vi "Labview_USB_I2C_AT24C02_SCTL.vi"() -> ()   [LabVIEW 2010]
uses:
  Labview_USB_I2C_AM2321B/lib/labview_32bit/ControlI2C/Ginkgo_Driver.dll
panel:
  out "Flag(T:read;F:write)":bool=TRUE
  in  "Constant":T1={"DevType"=1, "DevIndex"=0, "I2CIndex"=0, "Addr"=0, "SubAddr"=0}
  in  "pInitConfig":T2={"MasterMode"=1, "ControlMode"=1, "AddrType"=7, "SubAddrWidth"=0, "Addr"=0, "@dummy control@"=0, "@dummy control@"=0, "ClockSpeed"=0}
  in  "pTimeConfig":T3
  out "error out":errorcluster
  in  "Read":bool
  in  "Write":bool
  in  "Sub Addr(Hex)":u8 format="%x"
  in  "Slave Addr(Hex)":u8 format="%x"
  out "Read Data(Hex)":string
  in  "Channel Index":u16(ring) items=["0", "1"]
  in  "Speed":u32(ring)=800000 items=["800Kbps"=800000, "400Kbps"=400000, "200Kbps"=200000, "100Kbps"=100000, "50Kbps"=50000]
  in  "Write Data(Hex)":string
  in  "Device Index":u16(ring) items=["0", "1", "2", "3", "4", "5", "6", "7", "8", "9"]
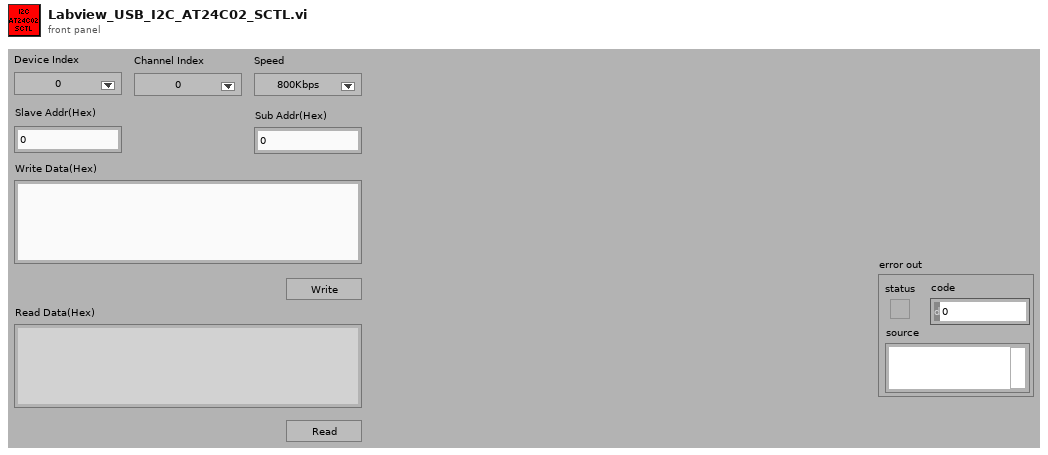
[diagram p1: front panel]
types:
  T1 = cluster{"DevType":i32, "DevIndex":i32, "I2CIndex":i32, "Addr":u16, "SubAddr":u32}
  T2 = cluster{"MasterMode":u8, "ControlMode":u8, "AddrType":u8, "SubAddrWidth":u8, "Addr":u16, "@dummy control@":i8, "@dummy control@":i8, "ClockSpeed":u32}
  T3 = cluster{"tHD_STA":u16, "tSU_STA":u16, "tLOW":u16, "tHIGH":u16, "tSU_DAT":u16, "tSU_STO":u16, "tDH":u16, "tDH_DAT":u16, "tAA":u16, "tR":u16, "tF":u16, "tBuf":u16, "tACK[0]":u8, "tACK[1]":u8, "tACK[2]":u8, "tACK[3]":u8, "tStart":u16, "tStop":u16}
  T4 = enum16{"Init", "Write", "Read", "Idel", "Close", "Error"}
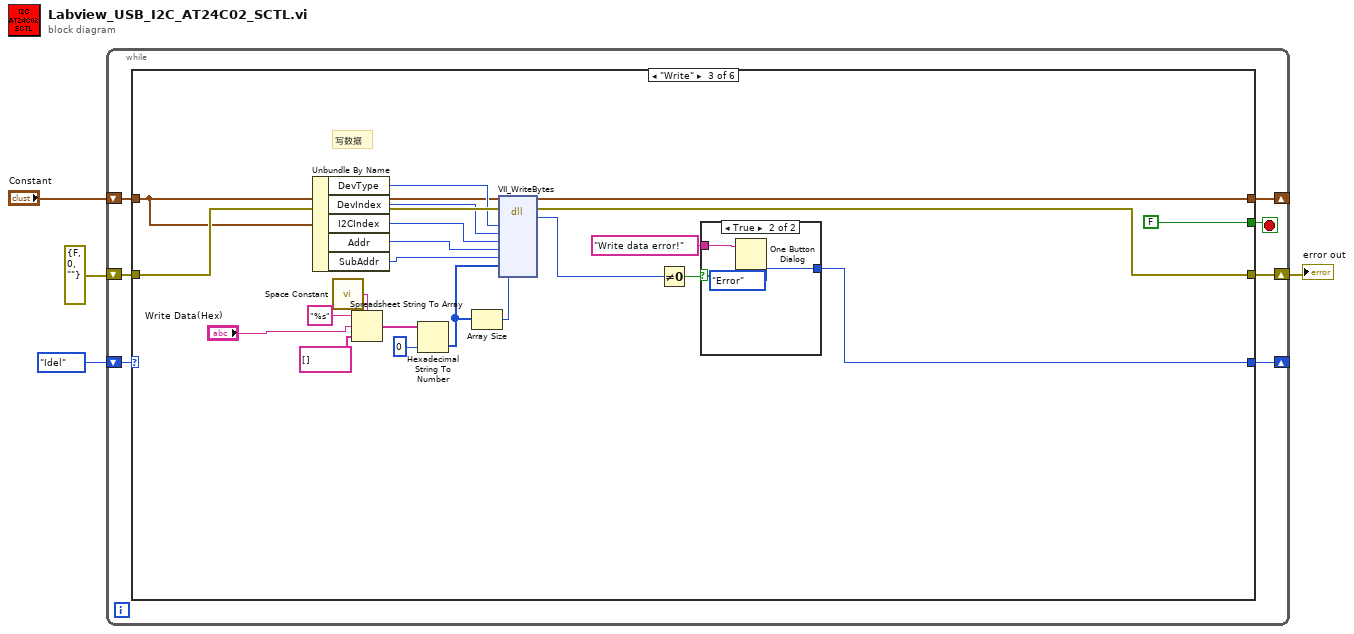
[diagram p0: block diagram]
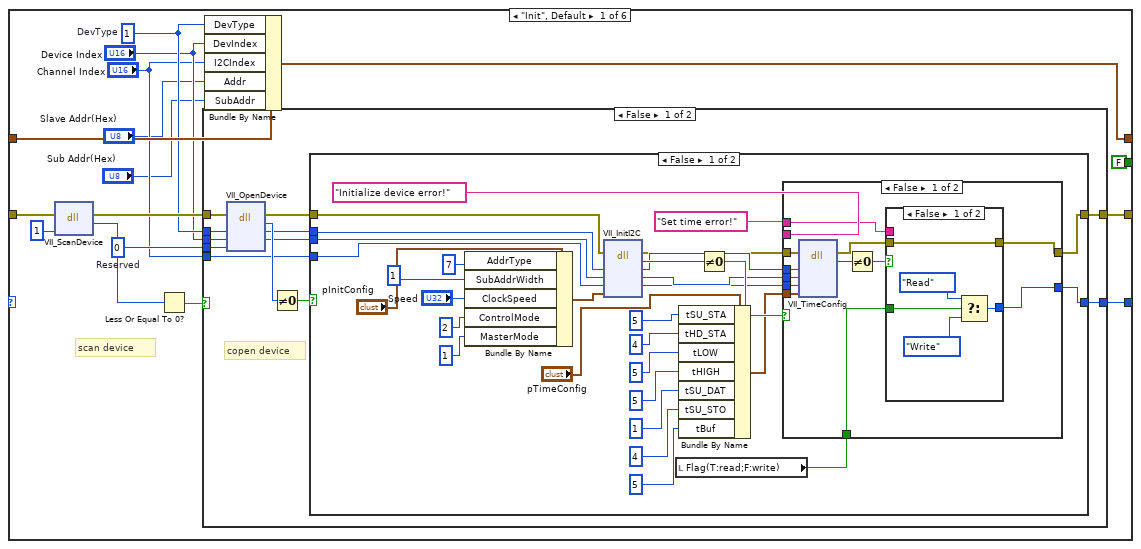
[diagram p2: hidden frame]
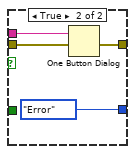
[diagram p3: hidden frame]
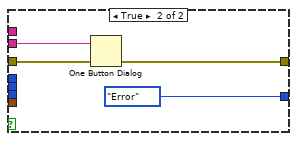
[diagram p4: hidden frame]
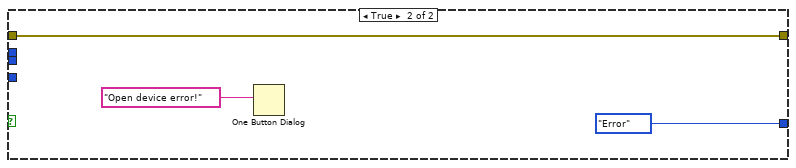
[diagram p5: hidden frame]
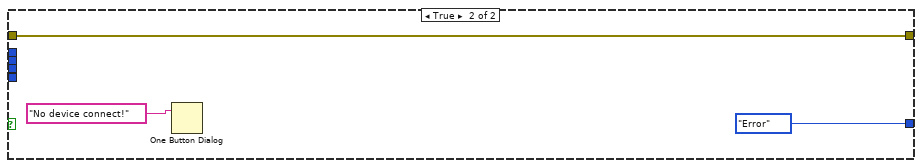
[diagram p6: hidden frame]
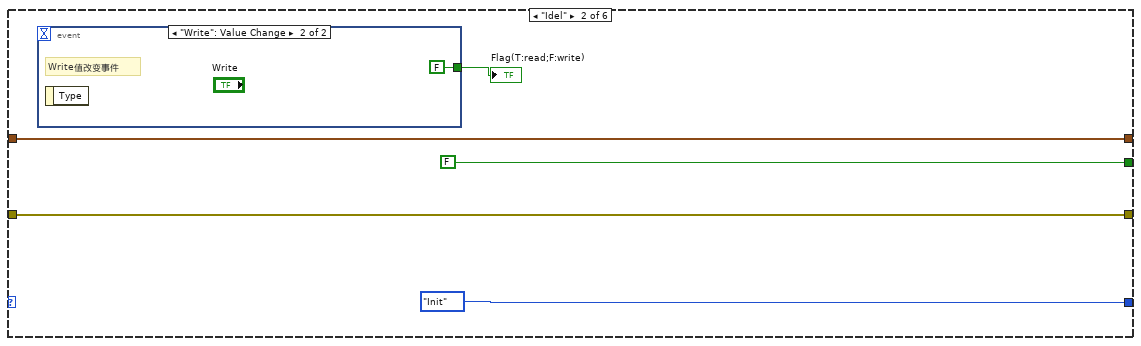
[diagram p7: hidden frame]
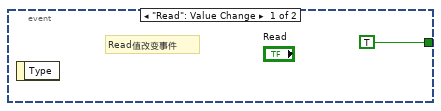
[diagram p8: hidden frame]
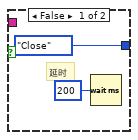
[diagram p9: hidden frame]
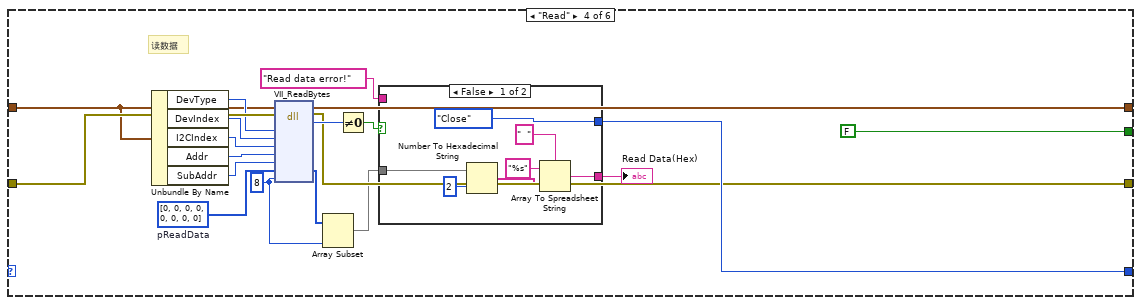
[diagram p10: hidden frame]
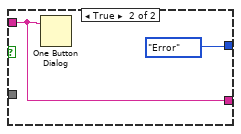
[diagram p11: hidden frame]
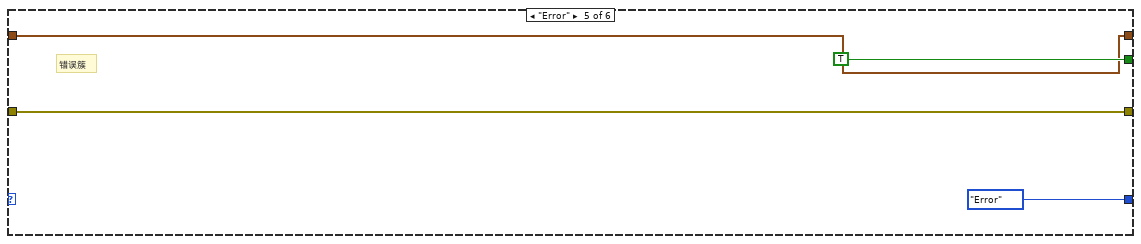
[diagram p12: hidden frame]
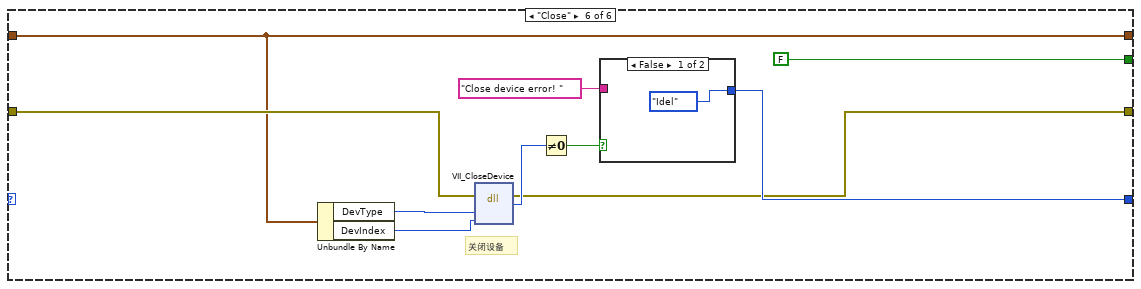
[diagram p13: hidden frame]
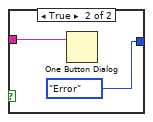
[diagram p14: hidden frame]
diagram:
  n1 = while {
    shift-right: [w11] -> _
    shift-left: T4."Idel" ("Enum") -> [w10]
    shift-right: [w8] -> w2
    shift-left: errorcluster {"status"=FALSE, "code"=0, "source"=""} ("error out") -> [w7]
    shift-right: [w5] -> _
    shift-left: "Constant" -> [w6]
    stop <- w9 stop-if-true
    n2 = case shown="\"Write\"" w10 {
      tunnel: [w19 T4."Init" ("Enum") w117 w140 T4."Error" ("Enum") w168] -> w11
      tunnel: [FALSE ("stop") FALSE ("stop") FALSE ("stop") FALSE ("stop") TRUE ("stop") FALSE ("stop")] -> w9
      tunnel: [w20 w103 w116 w139 w161 w167] -> w8
      tunnel: w7 -> [w21 w103 w126 w148 w161 w166]
      tunnel: w6 -> [w18 w102 w120 w138 w159 w165]
      tunnel: [w12 w102 w120 w138 w159 w165] -> w5
      frame "Init", Default {
        w22 = 0  # Reserved
        w17 = 1  # DevType
        # "scan device"
        n3 = dll-call lib="E:/Project/vt_ginkgo_examples/trunk/Labview/Ginkgo I2C/Labview_USB_I2C_AM2321B/lib/labview_32bit/ControlI2C/Ginkgo_Driver.dll" fn="VII_ScanDevice"(error in=w21, "NeedInit"=u8 1) -> (error out=w23:errorcluster, "return type"=w25:i32)  [unwired: 3 in, 1 out]
        n4 = Less Or Equal To 0?(x=w25) -> (x <= 0?=w24:bool)
        n5 = case shown="False" w24 {
          tunnel: [w33 T4."Error" ("Enum")] -> w19
          tunnel: w23 -> [w37 w98]
          tunnel: w22 -> [w36 _]
          tunnel: "Device Index" -> [w35 _]
          tunnel: w17 -> [w34 _]
          tunnel: [w29 w98] -> w20
          tunnel: "Channel Index" -> [w28 _]
          frame False {
            # "copen device"
            n6 = dll-call lib="E:/Project/vt_ginkgo_examples/trunk/Labview/Ginkgo I2C/Labview_USB_I2C_AM2321B/lib/labview_32bit/ControlI2C/Ginkgo_Driver.dll" fn="VII_OpenDevice"(error in=w37, "DevType"=w34, "DevIndex"=w35, "Reserved"=w36) -> (error out=w32:errorcluster, "return type"=w38:i32, "DevType"=w31:i32, "DevIndex"=w30:i32)  [unwired: 3 in, 1 out]
            n7 = Not Equal To 0?(x=w38) -> (x != 0?=w39:bool)
            n8 = case shown="False" w39 {
              tunnel: [w47 T4."Error" ("Enum")] -> w33
              tunnel: w32 -> [w50 w95]
              tunnel: w31 -> [w49 _]
              tunnel: w30 -> [w48 _]
              tunnel: [w46 w95] -> w29
              tunnel: w28 -> [w45 _]
              frame False {
                n9 = Bundle By Name(cluster="pInitConfig", "AddrType"=u8 7, "SubAddrWidth"=u8 1, "ClockSpeed"="Speed", "ControlMode"=u8 2, "MasterMode"=u8 1) -> (w68:T2)
                n10 = dll-call lib="E:/Project/vt_ginkgo_examples/trunk/Labview/Ginkgo I2C/Labview_USB_I2C_AM2321B/lib/labview_32bit/ControlI2C/Ginkgo_Driver.dll" fn="VII_InitI2C"(error in=w50, "DevType"=w49, "DevIndex"=w48, "I2CIndex"=w45, "pInitConfig"=w68) -> (error out=w62:errorcluster, "return type"=w70:i32, "DevType"=w65:i32, "DevIndex"=w64:i32, "I2CIndex"=w63:i32)  [unwired: 3 in, 1 out]
                n11 = local read "Flag(T:read;F:write)"() -> (w40:bool)
                n12 = Bundle By Name(cluster="pTimeConfig", "tSU_STA"=u16 5, "tHD_STA"=u16 4, "tLOW"=u16 5, "tHIGH"=u16 5, "tSU_DAT"=u16 1, "tSU_STO"=u16 4, "tBuf"=u16 5) -> (w53:T3)
                n13 = Not Equal To 0?(x=w70) -> (x != 0?=w69:bool)
                n14 = case shown="False" w69 {
                  tunnel: "Initialize device error!" ("message") -> [_ w93]
                  tunnel: [w74 T4."Error" ("Enum")] -> w47
                  tunnel: w65 -> [w82 _]
                  tunnel: w64 -> [w81 _]
                  tunnel: w63 -> [w80 _]
                  tunnel: w53 -> [w79 _]
                  tunnel: w62 -> [w78 w91]
                  tunnel: "Set time error!" ("message") -> [w75 _]
                  tunnel: [w71 w91] -> w46
                  tunnel: w40 -> [w73 _]
                  frame False {
                    n15 = dll-call lib="E:/Project/vt_ginkgo_examples/trunk/Labview/Ginkgo I2C/Labview_USB_I2C_AM2321B/lib/labview_32bit/ControlI2C/Ginkgo_Driver.dll" fn="VII_TimeConfig"(error in=w78, "DevType"=w82, "DevIndex"=w81, "I2CIndex"=w80, "pTimeConfig"=w79) -> (error out=w72:errorcluster, "return type"=w77:i32)  [unwired: 6 in, 1 out]
                    n16 = Not Equal To 0?(x=w77) -> (x != 0?=w76:bool)
                    n17 = case shown="False" w76 {
                      tunnel: w75 -> [_ w90]
                      tunnel: [w84 T4."Error" ("Enum")] -> w74
                      tunnel: w73 -> [w85 _]
                      tunnel: w72 -> [w83 w88]
                      tunnel: [w83 w88] -> w71
                      frame False {
                        n18 = Select(t=T4."Read" ("Enum"), s=w85, f=T4."Write" ("Enum")) -> (s? t:f=w84:T4)
                      }
                      frame True {
                        n19 = One Button Dialog(message=w90) -> ()  [unwired: 1 in, 1 out]
                      }
                    }
                  }
                  frame True {
                    n20 = One Button Dialog(message=w93) -> ()  [unwired: 1 in, 1 out]
                  }
                }
              }
              frame True {
                n21 = One Button Dialog(message="Open device error!") -> ()  [unwired: 1 in, 1 out]
              }
            }
          }
          frame True {
            n22 = One Button Dialog(message="No device connect!") -> ()  [unwired: 1 in, 1 out]
          }
        }
        n23 = Bundle By Name(cluster=w18, "DevType"=w17, "DevIndex"="Device Index", "I2CIndex"="Channel Index", "Addr"="Slave Addr(Hex)", "SubAddr"="Sub Addr(Hex)") -> (w12:T1)
      }
      frame "Idel" {
        n24 = event shown="[1] \"Write\": Value Change" {
          selector: _ -> [_ _]
          dyn-events: _ -> [_ _]
          timeout: _ -> [_ _]
          tunnel: [TRUE FALSE] -> w100
          event "Read": Value Change {
            # "Read值改变事件"
            n25 = event-data() -> ()  [unwired: 1 in, 1 out]
          }
          event "Write": Value Change {
            # "Write值改变事件"
            n26 = event-data() -> ()  [unwired: 1 in, 1 out]
          }
        }
        "Flag(T:read;F:write)" <- w100
      }
      frame "Write" {
        # "写数据"
        n27 = Unbundle By Name(w120) -> ("DevType"=w125:i32, "DevIndex"=w124:i32, "I2CIndex"=w123:i32, "Addr"=w122:u16, "SubAddr"=w121:u32)
        n28 = call <vilib>:"Space Constant.vi"() -> ("String"=w110:string)
        n29 = Spreadsheet String To Array(delimiter (Tab)=w110, format string="%s", spreadsheet string="Write Data(Hex)", array type (2D Dbl)=string[] []) -> (array=w113:string[])
        n30 = Hexadecimal String To Number(string=w113, default (0uL)=u8 0 ("default (0 U32)")) -> (number=w108:u8[])  [unwired: 1 in, 1 out]
        n31 = Array Size(array=w108) -> (size(s)=w107:i32)
        n32 = dll-call lib="E:/Project/vt_ginkgo_examples/trunk/Labview/Ginkgo I2C/Labview_USB_I2C_AM2321B/lib/labview_32bit/ControlI2C/Ginkgo_Driver.dll" fn="VII_WriteBytes"(error in=w126, "DevType"=w125, "DevIndex"=w124, "I2CIndex"=w123, "Addr"=w122, "SubAddr"=w121, "pWriteData"=w108, "Len"=w107) -> (error out=w116:errorcluster, "return type"=w118:i32)  [unwired: 9 in, 1 out]
        n33 = Not Equal To 0?(x=w118) -> (x != 0?=w115:bool)
        n34 = case shown="True" w115 {
          tunnel: "Write data error!" ("message") -> [_ w131]
          tunnel: [T4."Close" ("Enum") T4."Error" ("Enum")] -> w117
          frame False {
            # "延时"
            n35 = Wait (ms)(milliseconds to wait=u32 200) -> ()  [unwired: 1 out]
          }
          frame True {
            n36 = One Button Dialog(message=w131) -> ()  [unwired: 1 in, 1 out]
          }
        }
      }
      frame "Read" {
        w135 = u8[] [0, 0, 0, 0, 0, 0, 0, 0]  # pReadData
        w133 = u16 8 ("Len")
        # "读数据"
        n37 = Unbundle By Name(w138) -> ("DevType"=w147:i32, "DevIndex"=w146:i32, "I2CIndex"=w145:i32, "Addr"=w144:u16, "SubAddr"=w143:u32)
        n38 = dll-call lib="E:/Project/vt_ginkgo_examples/trunk/Labview/Ginkgo I2C/Labview_USB_I2C_AM2321B/lib/labview_32bit/ControlI2C/Ginkgo_Driver.*" fn="VII_ReadBytes"(error in=w148, "DevType"=w147, "DevIndex"=w146, "I2CIndex"=w145, "Addr"=w144, "SubAddr"=w143, "pReadData"=w135, "Len"=w133) -> (error out=w139:errorcluster, "return type"=w142:i32, "pReadData"=w134:u8[])  [unwired: 8 in, 1 out]
        n39 = Array Subset(array=w134, length=w133) -> (w132:u8[])  [unwired: 1 in]
        n40 = Not Equal To 0?(x=w142) -> (x != 0?=w137:bool)
        n41 = case shown="False" w137 {
          tunnel: "Read data error!" ("message") -> [_ w157]
          tunnel: [T4."Close" ("Enum") T4."Error" ("Enum")] -> w140
          tunnel: w132 -> [w151 _]
          tunnel: [w150 w157] -> w136
          frame False {
            n42 = Number To Hexadecimal String(1:i16 2 ("width (-)"), 2:w151) -> (0:w153:string[])
            n43 = Array To Spreadsheet String(delimiter (Tab)="  ", array=w153, 3:"%s" ("format string")) -> (spreadsheet string=w150:string)
          }
          frame True {
            n44 = One Button Dialog(message=w157) -> ()  [unwired: 1 in, 1 out]
          }
        }
        "Read Data(Hex)" <- w136
      }
      frame "Error" {
        # "错误簇"
      }
      frame "Close" {
        # "关闭设备"
        n45 = Unbundle By Name(w165) -> ("DevType"=w164:i32, "DevIndex"=w163:i32)
        n46 = dll-call lib="E:/Project/vt_ginkgo_examples/trunk/Labview/Ginkgo I2C/Labview_USB_I2C_AM2321B/lib/labview_32bit/ControlI2C/Ginkgo_Driver.dll" fn="VII_CloseDevice"(error in=w166, "DevType"=w164, "DevIndex"=w163) -> (error out=w167:errorcluster, "return type"=w170:i32)  [unwired: 4 in, 1 out]
        n47 = Not Equal To 0?(x=w170) -> (x != 0?=w169:bool)
        n48 = case shown="False" w169 {
          tunnel: "Close device error! " ("message") -> [_ w175]
          tunnel: [T4."Idel" ("Enum") T4."Error" ("Enum")] -> w168
          frame False {
          }
          frame True {
            n49 = One Button Dialog(message=w175) -> ()  [unwired: 1 in, 1 out]
          }
        }
      }
    }
  }
  "error out" <- w2
